vi "Start Transaction.vi"(8 "error in":errorcluster, 11 "DB-MySQL in":refnum<class "DB-MySQL.lvclass">) -> (0 "error out":errorcluster, 3 "DB-MySQL out":refnum<class "DB-MySQL.lvclass">)   [LabVIEW 2022 SP3, in "hse-db-mysql.lvlib" / "DB-MySQL.lvclass"]
doc: "Start a transaction to get sure all following SQL commands get executed or none.\n\n____\nHAMPEL SOFTWARE ENGINEERING v1.4.0 (2023-12-19 09:52)"
uses:
  DB-MySQL.lvclass
  DB-MySQL.lvclass/DB-MySQL.ctl
  <vilib>/Hampel Software Engineering/MySQLNetCom/MySQLNetCom.lvlib
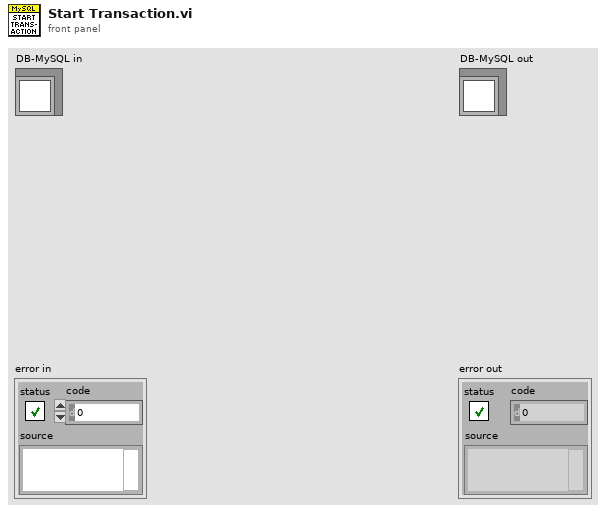
[diagram p1: front panel]
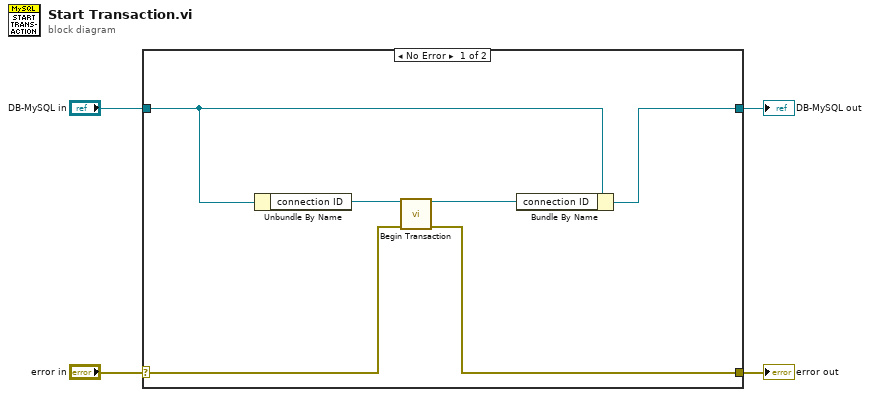
[diagram p0: block diagram]
diagram:
  n1 = case shown="No Error" "error in" {
    selector: "error in" -> [w6 w12]
    tunnel: [w5 w12] -> w3
    tunnel: [w9 w11] -> w1
    tunnel: "DB-MySQL in" -> [w10 w11]
    frame No Error {
      n2 = Unbundle By Name(w10) -> ("connection ID"=w8:refnum<k5>)
      n3 = call <vilib>:"Begin Transaction.vi"("connection ID in"=w8, "Error In"=w6) -> ("connection ID out"=w7:refnum<k5>, "Error Out"=w5:errorcluster)  [unwired: 12 in]
      n4 = Bundle By Name(cluster=w10, "connection ID"=w7) -> (w9:refnum<class "DB-MySQL.lvclass">)
    }
    frame Error {
    }
  }
  "error out" <- w3
  "DB-MySQL out" <- w1
